vi "load user configuration.vi"() -> (1 "RT config file path":path, 3 "config parameters":T13 {"messageHandler"."params"."controlChannels"."ballControl" items=["Module6/output0", "Module6/output1", "Module6/output2", "Module6/output3", "Not-Used"]; "messageHandler"."params"."controlChannels"."butterflyControl" items=["Module6/output0", "Module6/output1", "Module6/output2", "Module6/output3", "Not-Used"]; "messageHandler"."params"."controlChannels"."speedControl" items=["Module6/output0", "Module6/output1", "Module6/output2", "Module6/output3", "Not-Used"]})   [LabVIEW 2018]
uses:
  type defs/message handler data.ctl
  customVI/liveData/state.ctl
  type defs/comms loop data.ctl
  ICL-LabVIEW_General/Incident logger/Incident logger.lvclass
  <vilib>/Modbus/master/Modbus Master.lvclass
  type defs/data stream data.ctl
  type defs/data processor data.ctl
  type defs/channelLimitControl.ctl
  type defs/limitActions.ctl
  type defs/file IO data.ctl
  type defs/channelControl.ctl
  RT/Type Defs/channelScalingTypes.ctl
  RT/Type Defs/scalingMethods.ctl
  ICL-LabVIEW_General/data channels/parent class/Data Channel.lvclass
  type defs/UI loop data.ctl
  type defs/error messages data.ctl
  <vilib>/Utility/config.llb/Read Key (Path).vi
  <vilib>/Utility/config.llb/Read Key (U32).vi
  <vilib>/Utility/config.llb/Read Key (Boolean).vi
  <vilib>/Utility/config.llb/Read Key (Double).vi
  <vilib>/Utility/config.llb/Read Key (String).vi
  <vilib>/Utility/config.llb/NI_LVConfig.lvlib
panel:
  out "Default parameters":string[](array[string])
  out "unmatched parameters":string[](array[string])
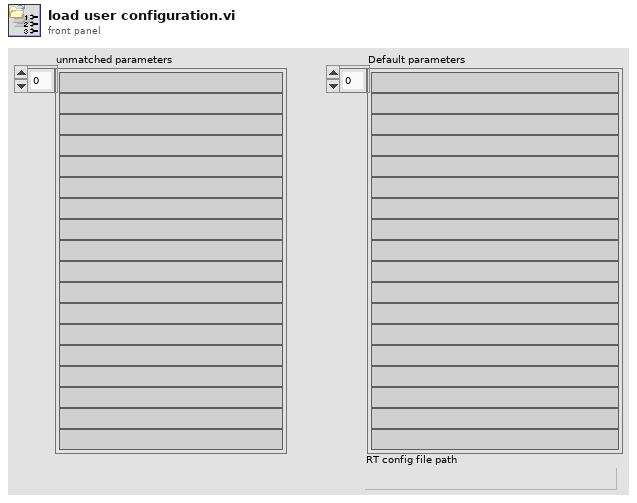
[diagram p1: front panel]
types:
  T1 = typedef "message handler data.ctl" = cluster{"params":cluster{"configFileID":u32, "configFilePath":path, "channelConfigFilePath":path, "incidentLogfile":path, "controlChannels":cluster{"ballControl":u16, "butterflyControl":u16, "speedControl":u16}, "pulsatorVIPath":path, "customVIPath":path, "HowdenAir":cluster{"vent Howden":bool, "Howden%":dbl}}, "vars":cluster{"commsStatus":bool[], "controlIndex":cluster{"ballControl":u16, "butterflyControl":u16, "speedControl":u16}, "customVIRef":refnum<vi>, "Interlocks":cluster{"gearboxOil":bool, "bearingOil":bool, "gearboxAir":bool}, "motorRunning":bool, "liveDataQ":refnum<queue>[]}}
  T2 = typedef "comms loop data.ctl" = cluster{"params":cluster{"commandStream":cluster{"reader name":string, "writer name":string, "stream buffer size":i32}, "errorStream":cluster{"reader name":string, "writer name":string, "stream buffer size":i32}, "RT IP address":string, "pulserControllerIP":string}, "vars":cluster{"commandStream":refnum<k21>, "Incident logger":refnum<class "Incident logger.lvclass">, "check error scheduled message":u32, "errorStream":refnum<k21>, "watchdogScheduleID":u32, "pulsator":cluster{"pulser connection":refnum<class "Modbus Master.lvclass">, "pulserConnected":bool, "pulsatorScheduleID":u32, "pulserRunning":bool}}}
  T3 = typedef "data stream data.ctl" = cluster{"params":cluster{"Stream":cluster{"reader name":string, "RT IP address":string, "writer name":string, "stream buffer size":i32}}, "vars":cluster{"data stream":refnum<k21>}}
  T4 = typedef "data processor data.ctl" = cluster{"params":cluster{"controlFeedback":cluster{"butterflyValue":u16, "ballValue":u16, "massflow":u16, "pressureRatio":u16, "compSpeed":u16}, "DAQrate":enum16{"50 kHz", "25 kHz", "16.6 kHz", "12.5 kHz", "10 kHz", "8.33 kHz", "7.14 kHz", "6.25 kHz", "5.55 kHz", "5 kHz"}, "safetyChannels":cluster{"oilP":u16, "airP":u16, "water":u16, "channelLimit":T5[]}, "channelConfigPath":path}, "vars":cluster{"controlFeedback":cluster{"butterflyValue":u16, "ballValue":u16, "massflow":u16, "pressureRatio":u16, "compSpeed":u16}, "activeChannelNames":string[], "activeChannelUnits":string[], "offset trigger":bool, "offsets":dbl[], "activeChannelLimitIndex":u16[], "liveData":bool}}
  T5 = typedef "channelLimitControl.ctl" = cluster{"channelID":u16, "Enabled":bool, "warnValue":dbl, "limitValue":dbl, "Invert":bool, "limitAction":T6}
  T6 = typedef "limitActions.ctl" = enum16{"stop", "shutdown", "ignore"}
  T7 = typedef "file IO data.ctl" = cluster{"params":cluster{"startFolder":path, "channelConfigPath":path}, "vars":cluster{"channelConfig ":T8[], "writing":cluster{"streaming":bool, "fixedLength":bool, "pointCount":u32, "timeZero":dbl, "pointsWritten":u32, "dataRate":u16}, "channelCount":u16, "fileTarget":cluster{"Save folder":path, "Target filename":string, "file ref":refnum<file>, "pulsatorSpeed":string, "motorSpeed":string, "valvePosition":string, "torqueFilter":bool, "pulsatorRunning":bool, "motorRunning":bool}, "channels":refnum<class "Data Channel.lvclass">[]}}
  T8 = typedef "channelControl.ctl" = cluster{"index":u16, "active":bool, "channelType":T9, "module":u16, "terminal":u16, "channelName":string, "scalingMethod":T10, "scalingParameters":dbl[], "scaledUnits":string, "tempOffset":dbl}
  T9 = typedef "channelScalingTypes.ctl" = enum16{"calculation", "measurement", "scanivalve", "output", "digital"}
  T10 = typedef "scalingMethods.ctl" = enum16{"none", "linear", "thermocouple", "polynomial", "encoder", "RTD"}
  T11 = typedef "UI loop data.ctl" = cluster{"params":cluster{"channelConfigPath":path, "version":string}, "vars":cluster{"tempOffsets":dbl[], "encoderFallingEdge":bool, "controlRefs":cluster{"mainVI":refnum<vi>, "menu":refnum<k9>, "motorStart":refnum<vi>, "butterfly":refnum<vi>, "ball":refnum<vi>, "speed":refnum<vi>, "logLimit":refnum<vi>, "pointLimit":refnum<vi>, "logData":refnum<vi>}}}
  T12 = typedef "error messages data.ctl" = cluster{"params":cluster{"eg":bool}, "vars":cluster{"eg":bool}}
  T13 = cluster{"messageHandler":T1, "comms":T2, "dataStream":T3, "dataProcessor":T4, "fileIO":T7, "userInterface":T11, "errors":T12}
  T14 = typedef "NI_LVConfig.lvlib/Config Data RefNum.ctl" = refnum<k1>
  T15 = typedef "Message loop data.ctl" = cluster{"Parameters":cluster{"FPGA Ref":T16, "configID":u32, "activeChannels":cluster{"index":u16, "name":string}[]}, "Variables":cluster{"RT Status":T17, "watchdog":timestamp, "limitsEnabled":bool, "Interlocks":cluster{"gearboxOil":bool, "bearingOil":bool, "gearboxAir":bool}}}
  T16 = typedef "FPGA reference.ctl" = refnum<k20>
  T17 = typedef "RT Status.ctl" = cluster{"Comms loop":bool, "scheduler loop":bool, "data process loop":bool, "FIFO loop":bool, "Command Stream":bool, "Error Stream":bool, "FPGA FIFO":bool, "Data Stream":bool}
  T18 = typedef "Analogue loop data.ctl" = cluster{"Params":cluster{"FPGA ref":T16, "Total Channels":u32}, "Variables":cluster{"FIFO wait counter":u16, "FIFO read trigger":u32}}
  T19 = typedef "comms data.ctl" = cluster{"Parameters":cluster{"error writer name":string, "command reader name":string, "error buffer size":i32, "command buffer size":i32, "scanivalveIP":string, "scanivalvePeriod":u16}, "Variables":cluster{"listen schedule":u32, "incident buffer":T20[], "command stream":refnum<k21>, "error stream":refnum<k21>, "waiting for command stream connect":bool, "waiting for error stream connect":bool, "scanivalve connection":refnum<k5>, "scanivalveScheduleID":u32, "activeScanivalvePorts":i32[], "channelCount":i16}, "scanivalveConfig":T21}
  T20 = typedef "generic incident.ctl" = cluster{"timestamp":timestamp, "type":string, "Variant":variant}
  T21 = typedef "Scanivalve API.lvlib/scanivalveConfig.ctl" = cluster{"listS":T22, "listC":T23, "listSG":T24, "activeChannels":T25}
  T22 = typedef "Scanivalve API.lvlib/listS.ctl" = cluster{"period":u16, "ADtrig":bool, "ScanTrig":bool, "page":u16, "qpkts":u16}
  T23 = typedef "Scanivalve API.lvlib/listC.ctl" = cluster{"ZC":bool, "unitScan":string, "CvtUnit":dbl, "bin":bool, "EU":bool}
  T24 = typedef "Scanivalve API.lvlib/listSG.ctl" = cluster{"Avg1":u16, "FPS1":u16, "SGEnable1":bool}
  T25 = typedef "Scanivalve API.lvlib/chan1.ctl" = cluster{"Chan1":cluster{"101":bool, "102":bool, "103":bool, "104":bool, "109":bool, "110":bool, "111":bool, "112":bool, "201":bool, "202":bool, "203":bool, "204":bool, "209":bool, "210":bool, "211":bool, "212":bool, "301":bool, "302":bool, "303":bool, "304":bool, "309":bool, "310":bool, "311":bool, "312":bool, "401":bool, "402":bool, "403":bool, "404":bool, "409":bool, "410":bool, "411":bool, "412":bool}}
  T26 = typedef "Data processing loop data.ctl" = cluster{"Parameters":cluster{"FPGA Ref":T16, "data stream":cluster{"data writer name":string, "NS write buffer size":i32, "NS Buffer length":u32}, "FIFO Depth":u32, "Channel controls":cluster{"FIFO channel count":i32, "active indices":i16[], "active channels":i32, "channelScaling":T8[], "scanivalveCount":i32, "channels":refnum<class "Data Channel.lvclass">[]}, "safetyChannels":cluster{"oilP":u16, "airP":u16, "water":u16, "channelLimits":T5[]}, "speedChannel":i32, "maxSpeedLimit":dbl, "Torque":cluster{"fixedOffset":dbl, "filter":bool, "fallingEdge":bool, "swapEncoders":bool}}, "Variables":cluster{"Intermediary buffer":dbl[][], "buffer position":u32, "write loop counter":u16, "NS write trigger":u32, "NS Connection status":bool, "waiting for NS":bool, "labAmbient":cluster{"pressure":dbl, "temperature":dbl}, "scanivalvePorts":u16[], "scanivalvePressures":dbl[], "data stream":refnum<k21>, "activeChannelLimitIndex":u16[], "runningSpeedLimit":dbl, "speedChannelIndex":i32, "Interlocks":cluster{"gearboxOil":bool, "bearingOil":bool, "gearboxAir":bool}, "interlockChannels":cluster{"gearboxOil":i32, "bearingOil":i32, "air":i32}, "limitStates":cluster{"warn":bool, "alarm":bool}[]}}
  T27 = cluster{"Message":T15, "FIFO":T18, "Comms data":T19, "Data processor":T26}
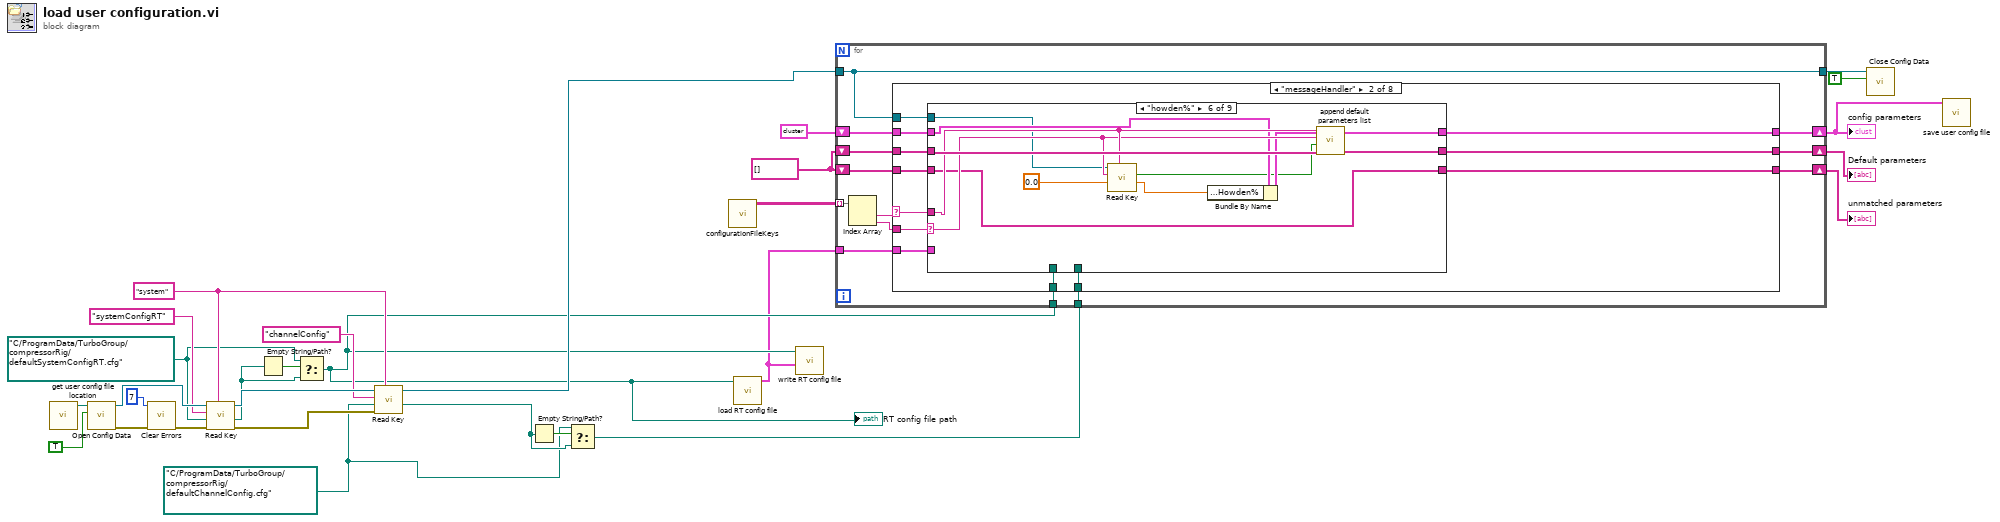
[diagram p0: block diagram]
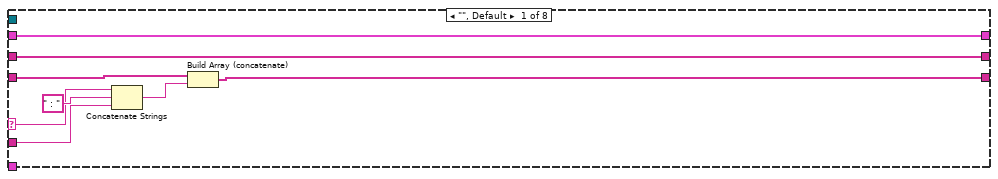
[diagram p2: hidden frame]
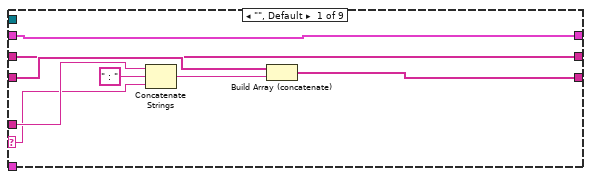
[diagram p3: hidden frame]
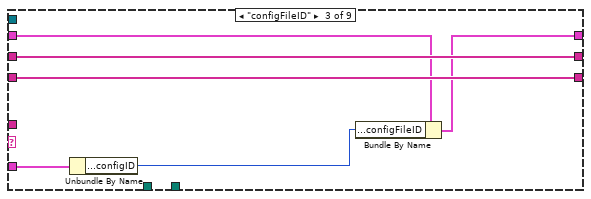
[diagram p5: hidden frame]
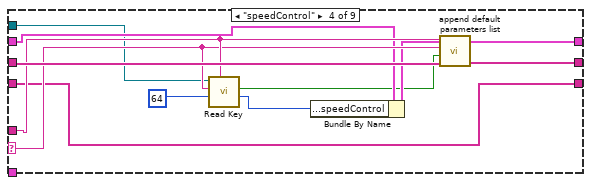
[diagram p6: hidden frame]
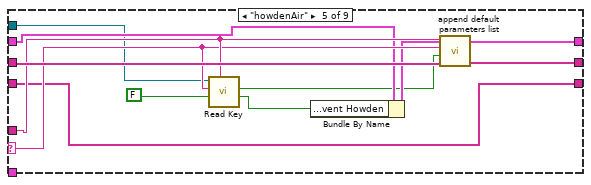
[diagram p7: hidden frame]
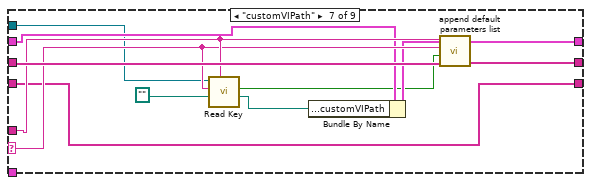
[diagram p8: hidden frame]
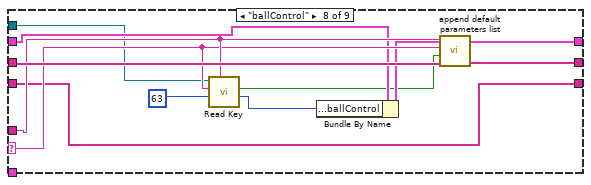
[diagram p9: hidden frame]
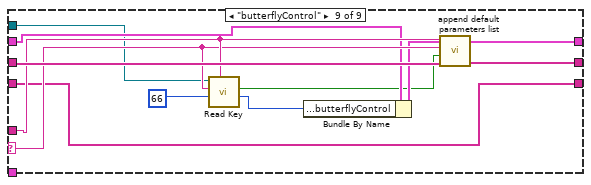
[diagram p10: hidden frame]
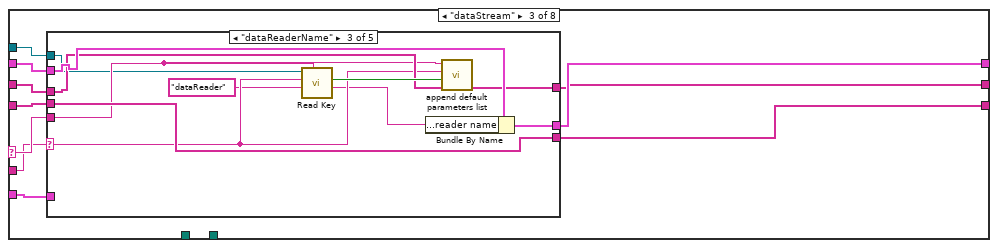
[diagram p11: hidden frame]
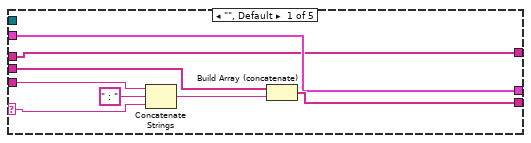
[diagram p12: hidden frame]
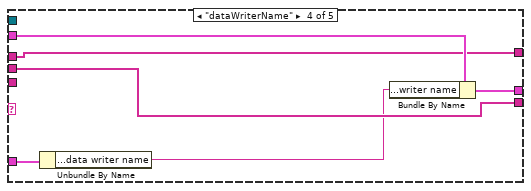
[diagram p14: hidden frame]
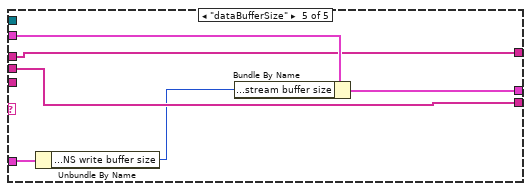
[diagram p15: hidden frame]
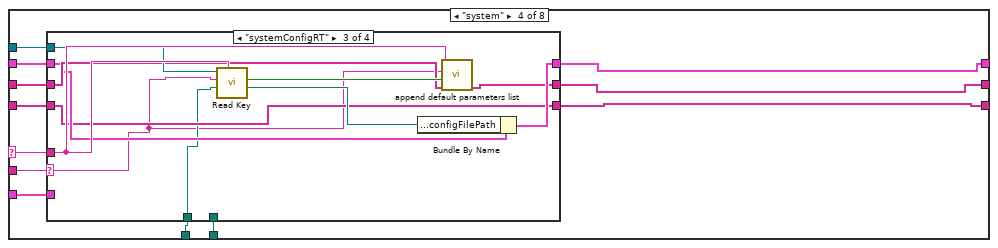
[diagram p16: hidden frame]
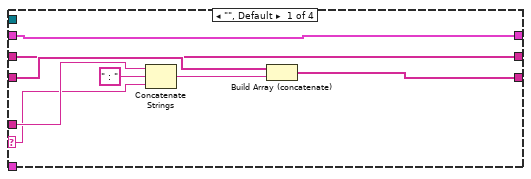
[diagram p17: hidden frame]
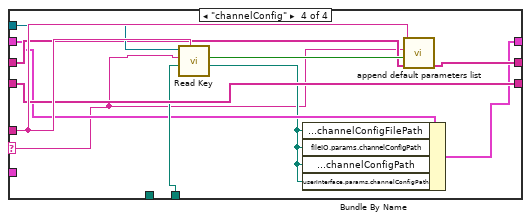
[diagram p19: hidden frame]
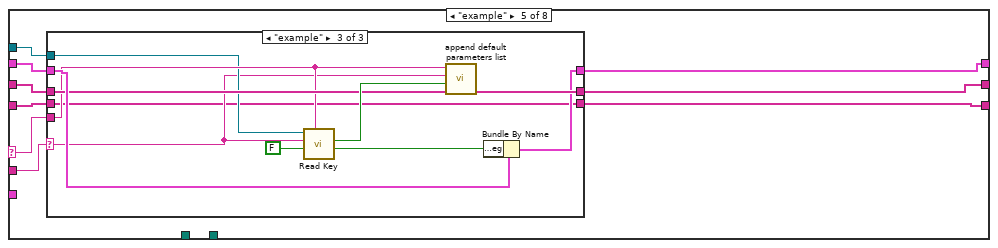
[diagram p20: hidden frame]
diagram:
  w20 = string[] []
  w4 = path "C:/ProgramData/TurboGroup/compressorRig/defaultChannelConfig.cfg" ("default value")
  w7 = path "C:/ProgramData/TurboGroup/compressorRig/defaultSystemConfigRT.cfg" ("default value")
  w23 = "system" ("section")
  n1 = call "get user config file location.vi"() -> ("userConfigPath"=w29:path)  [unwired: 11 in]
  n2 = call <vilib>:"Open Config Data.vi"("create file if necessary (T)"=TRUE, "configuration file path"=w29) -> ("error out"=w27:errorcluster, "refnum"=w28:T14)  [unwired: 7 in, 1 out]
  n3 = call <vilib>:"Clear Errors.vi"("error in (no error)"=w27, "specific error code to clear (0: all)"=7) -> ("error out"=w14:errorcluster)  [unwired: 4 in, 1 out]
  n4 = call-poly <vilib>:"Read Key.vi"("section"=w23, "error in (no error)"=w14, "default value"=w7, "key"="systemConfigRT", "refnum"=w28) -> ("error out"=w24:errorcluster, "value"=w8:path, "refnum out"=w25:T14)  [unwired: 3 in, 1 out]
  n5 = Empty String/Path?(string/path=w8) -> (empty?=w9:bool)
  n6 = Select(t=w7, s=w9, f=w8) -> (s? t:f=w2:path)
  "RT config file path" <- w2
  n7 = call-poly <vilib>:"Read Key.vi"("section"=w23, "error in (no error)"=w24, "default value"=w4, "key"="channelConfig", "refnum"=w25) -> ("value"=w5:path, "refnum out"=w18:T14)  [unwired: 3 in, 2 out]
  n8 = Empty String/Path?(string/path=w5) -> (empty?=w6:bool)
  n9 = Select(t=w4, s=w6, f=w5) -> (s? t:f=w3:path)
  n10 = call "configurationFileKeys.vi"() -> ("userConfigKeys"=w16:string[][])  [unwired: 9 in, 2 out]
  n11 = call "load RT config file.vi"("configuration file path (RT local)"=w2) -> ("config data out"=w1:T27)  [unwired: 7 in, 3 out]
  n12 = call "write RT config file.vi"("RT config"=w1, "RT config file path"=w2) -> ()  [unwired: 10 in]
  n13 = for {
    shift-right: [w41] -> w21
    shift-left: w20 -> [w42]
    shift-right: [w39] -> w10
    shift-left: T13 {"messageHandler"={"params"={"configFileID"=0, "configFilePath"=path "", "channelConfigFilePath"=path "", "incidentLogfile"=path "", "controlChannels"={"ballControl"=0, "butterflyControl"=0, "speedControl"=0}, "pulsatorVIPath"=path "", "customVIPath"=path "", "HowdenAir"={"vent Howden"=FALSE, "Howden%"=0.0}}, "vars"={"commsStatus"=[], "controlIndex"={"ballControl"=0, "butterflyControl"=0, "speedControl"=0}, "customVIRef"=refnum, "Interlocks"={"gearboxOil"=FALSE, "bearingOil"=FALSE, "gearboxAir"=FALSE}, "motorRunning"=FALSE, "liveDataQ"=[]}}, "comms"={"params"={"commandStream"={"reader name"="", "writer name"="", "stream buffer size"=0}, "errorStream"={"reader name"="", "writer name"="", "stream buffer size"=0}, "RT IP address"="", "pulserControllerIP"=""}, "vars"={"commandStream"="", "Incident logger"=refnum, "check error scheduled message"=0, "errorStream"="", "watchdogScheduleID"=0, "pulsator"={"pulser connection"=refnum, "pulserConnected"=FALSE, "pulsatorScheduleID"=0, "pulserRunning"=FALSE}}}, "dataStream"={"params"={"Stream"={"reader name"="", "RT IP address"="", "writer name"="", "stream buffer size"=0}}, "vars"={"data stream"=""}}, "dataProcessor"={"params"={"controlFeedback"={"butterflyValue"=0, "ballValue"=0, "massflow"=0, "pressureRatio"=0, "compSpeed"=0}, "DAQrate"=enum."50 kHz", "safetyChannels"={"oilP"=0, "airP"=0, "water"=0, "channelLimit"=[]}, "channelConfigPath"=path ""}, "vars"={"controlFeedback"={"butterflyValue"=0, "ballValue"=0, "massflow"=0, "pressureRatio"=0, "compSpeed"=0}, "activeChannelNames"=[], "activeChannelUnits"=[], "offset trigger"=FALSE, "offsets"=[], "activeChannelLimitIndex"=[], "liveData"=FALSE}}, "fileIO"={"params"={"startFolder"=path "", "channelConfigPath"=path ""}, "vars"={"channelConfig "=[], "writing"={"streaming"=FALSE, "fixedLength"=FALSE, "pointCount"=0, "timeZero"=0.0, "pointsWritten"=0, "dataRate"=0}, "channelCount"=0, "fileTarget"={"Save folder"=path "", "Target filename"="", "file ref"=refnum, "pulsatorSpeed"="", "motorSpeed"="", "valvePosition"="", "torqueFilter"=FALSE, "pulsatorRunning"=FALSE, "motorRunning"=FALSE}, "channels"=[]}}, "userInterface"={"params"={"channelConfigPath"=path "", "version"=""}, "vars"={"tempOffsets"=[], "encoderFallingEdge"=FALSE, "controlRefs"={"mainVI"=refnum, "menu"=refnum, "motorStart"=refnum, "butterfly"=refnum, "ball"=refnum, "speed"=refnum, "logLimit"=refnum, "pointLimit"=refnum, "logData"=refnum}}}, "errors"={"params"={"eg"=FALSE}, "vars"={"eg"=FALSE}}} ("parameters") -> [w40]
    tunnel: w18 -> [w33]
    tunnel: w16 -> [w38] mode=indexing
    shift-right: [w35] -> w19
    shift-left: w20 -> [w34]
    tunnel: [w33] -> w15
    tunnel: w1 -> [w32]
    tunnel: w2 -> [w31]
    tunnel: w3 -> [w30]
    n14 = Index Array(array=w38) -> (element #1=w37:string, element #2=w36:string)  [unwired: 2 in]
    n15 = case shown="\"messageHandler\"" w37 {
      selector: w37 -> [w46 w61 w154 w194 w242 w273 w370 w402]
      tunnel: w42 -> [w48 w62 w155 w198 w243 w274 w371 w403]
      tunnel: [w47 w60 w153 w196 w241 w272 w369 w401] -> w41
      tunnel: w40 -> [w45 w58 w151 w200 w239 w270 w367 w400]
      tunnel: [w45 w59 w152 w201 w240 w271 w368 w399] -> w39
      tunnel: w33 -> [_ w54 w147 w195 w235 w266 w363 w398]
      tunnel: w36 -> [w44 w57 w150 w193 w238 w269 w366 w397]
      tunnel: [w43 w56 w149 w197 w237 w268 w365 w395] -> w35
      tunnel: w34 -> [w43 w55 w148 w199 w236 w267 w364 w396]
      tunnel: w32 -> [_ w53 w146 w192 _ _ _ w394]
      tunnel: w31 -> [_ w52 _ w191 _ _ _ _]
      tunnel: w30 -> [_ w51 _ w190 _ _ _ _]
      frame "", Default {
        n16 = Concatenate Strings(w46, " : " ("string"), w44) -> (w49:string)
        n17 = Build Array (concatenate)(w48, w49) -> (w47:string[])
      }
      frame "messageHandler" {
        n18 = case shown="\"howden%\"" w57 {
          selector: w57 -> [w68 _ _ w87 w98 w109 w120 w131 w142]
          tunnel: w62 -> [w70 w73 w79 w84 w96 w107 w118 w128 w139]
          tunnel: w61 -> [w69 _ _ w88 w99 w110 w121 w132 w143]
          tunnel: [w65 w73 w79 w84 w96 w107 w118 w128 w139] -> w60
          tunnel: [w64 w72 w75 w83 w95 w106 w117 w127 w138] -> w59
          tunnel: w58 -> [w64 w72 w76 w85 w97 w108 w119 w129 w140]
          tunnel: [w63 w71 w78 w90 w101 w112 w123 w134 w145] -> w56
          tunnel: w55 -> [w63 w71 w78 w89 w100 w111 w122 w133 w144]
          tunnel: w54 -> [_ _ _ w80 w92 w103 w114 w124 w135]
          tunnel: w53 -> [_ _ w77 _ _ _ _ _ _]
          tunnel: w52 -> [_ _ _ _ _ _ _ _ _]
          tunnel: w51 -> [_ _ _ _ _ _ _ _ _]
          frame "", Default {
            n19 = Concatenate Strings(w69, " : " ("string"), w68) -> (w66:string)
            n20 = Build Array (concatenate)(w70, w66) -> (w65:string[])
          }
          frame "none" {
          }
          frame "configFileID" {
            n21 = Unbundle By Name(w77) -> ("Message.Parameters.configID"=w74:u32)
            n22 = Bundle By Name(cluster=w76, "messageHandler.params.configFileID"=w74) -> (w75:T13)
          }
          frame "speedControl" {
            n23 = call-poly <vilib>:"Read Key.vi"("section"=w88, "default value"=u16 64, "key"=w87, "refnum"=w80) -> ("value"=w82:u32, "found?"=w81:bool)  [unwired: 4 in, 2 out]
            n24 = Bundle By Name(cluster=w85, "messageHandler.params.controlChannels.speedControl"=w82) -> (w83:T13)
            n25 = call "append default parameters list.vi"("default parameters in"=w89, "parameter found?"=w81, "Key"=w87, "Section"=w88) -> ("default parameters out"=w90:string[])  [unwired: 7 in]
          }
          frame "howdenAir" {
            n26 = call-poly <vilib>:"Read Key.vi"("section"=w99, "default value"=FALSE, "key"=w98, "refnum"=w92) -> ("value"=w94:bool, "found?"=w93:bool)  [unwired: 4 in, 2 out]
            n27 = Bundle By Name(cluster=w97, "messageHandler.params.HowdenAir.vent Howden"=w94) -> (w95:T13)
            n28 = call "append default parameters list.vi"("default parameters in"=w100, "parameter found?"=w93, "Key"=w98, "Section"=w99) -> ("default parameters out"=w101:string[])  [unwired: 7 in]
          }
          frame "howden%" {
            n29 = call-poly <vilib>:"Read Key.vi"("section"=w110, "default value"=0.0, "key"=w109, "refnum"=w103) -> ("value"=w105:dbl, "found?"=w104:bool)  [unwired: 4 in, 2 out]
            n30 = Bundle By Name(cluster=w108, "messageHandler.params.HowdenAir.Howden%"=w105) -> (w106:T13)
            n31 = call "append default parameters list.vi"("default parameters in"=w111, "parameter found?"=w104, "Key"=w109, "Section"=w110) -> ("default parameters out"=w112:string[])  [unwired: 7 in]
          }
          frame "customVIPath" {
            n32 = call-poly <vilib>:"Read Key.vi"("section"=w121, "default value"=path "", "key"=w120, "refnum"=w114) -> ("value"=w116:path, "found?"=w115:bool)  [unwired: 4 in, 2 out]
            n33 = Bundle By Name(cluster=w119, "messageHandler.params.customVIPath"=w116) -> (w117:T13)
            n34 = call "append default parameters list.vi"("default parameters in"=w122, "parameter found?"=w115, "Key"=w120, "Section"=w121) -> ("default parameters out"=w123:string[])  [unwired: 7 in]
          }
          frame "ballControl" {
            n35 = call-poly <vilib>:"Read Key.vi"("section"=w132, "default value"=u16 63, "key"=w131, "refnum"=w124) -> ("value"=w126:u32, "found?"=w125:bool)  [unwired: 4 in, 2 out]
            n36 = Bundle By Name(cluster=w129, "messageHandler.params.controlChannels.ballControl"=w126) -> (w127:T13)
            n37 = call "append default parameters list.vi"("default parameters in"=w133, "parameter found?"=w125, "Key"=w131, "Section"=w132) -> ("default parameters out"=w134:string[])  [unwired: 7 in]
          }
          frame "butterflyControl" {
            n38 = call-poly <vilib>:"Read Key.vi"("section"=w143, "default value"=u16 66, "key"=w142, "refnum"=w135) -> ("value"=w137:u32, "found?"=w136:bool)  [unwired: 4 in, 2 out]
            n39 = Bundle By Name(cluster=w140, "messageHandler.params.controlChannels.butterflyControl"=w137) -> (w138:T13)
            n40 = call "append default parameters list.vi"("default parameters in"=w144, "parameter found?"=w136, "Key"=w142, "Section"=w143) -> ("default parameters out"=w145:string[])  [unwired: 7 in]
          }
        }
      }
      frame "dataStream" {
        n41 = case shown="\"dataReaderName\"" w150 {
          selector: w150 -> [w161 _ w170 _ _]
          tunnel: w155 -> [w163 w166 w177 w183 w189]
          tunnel: w154 -> [w162 _ w171 _ _]
          tunnel: [w158 w166 w177 w183 w189] -> w153
          tunnel: [w157 w165 w175 w181 w187] -> w152
          tunnel: w151 -> [w157 w165 w176 w182 w188]
          tunnel: [w156 w164 w172 w178 w184] -> w149
          tunnel: w148 -> [w156 w164 w173 w178 w184]
          tunnel: w147 -> [_ _ w169 _ _]
          tunnel: w146 -> [_ _ _ w180 w186]
          frame "", Default {
            n42 = Concatenate Strings(w162, " : " ("string"), w161) -> (w159:string)
            n43 = Build Array (concatenate)(w163, w159) -> (w158:string[])
          }
          frame "none" {
          }
          frame "dataReaderName" {
            n44 = call-poly <vilib>:"Read Key.vi"("section"=w171, "default value"="dataReader" ("name or relative path"), "key"=w170, "refnum"=w169) -> ("value"=w167:string, "found?"=w174:bool)  [unwired: 4 in, 2 out]
            n45 = Bundle By Name(cluster=w176, "dataStream.params.Stream.reader name"=w167) -> (w175:T13)
            n46 = call "append default parameters list.vi"("default parameters in"=w173, "parameter found?"=w174, "Key"=w170, "Section"=w171) -> ("default parameters out"=w172:string[])  [unwired: 7 in]
          }
          frame "dataWriterName" {
            n47 = Unbundle By Name(w180) -> ("Data processor.Parameters.data stream.data writer name"=w179:string)
            n48 = Bundle By Name(cluster=w182, "dataStream.params.Stream.writer name"=w179) -> (w181:T13)
          }
          frame "dataBufferSize" {
            n49 = Unbundle By Name(w186) -> ("Data processor.Parameters.data stream.NS write buffer size"=w185:i32)
            n50 = Bundle By Name(cluster=w188, "dataStream.params.Stream.stream buffer size"=w185) -> (w187:T13)
          }
        }
      }
      frame "system" {
        n51 = case shown="\"systemConfigRT\"" w193 {
          selector: w193 -> [w207 _ w213 w224]
          tunnel: w198 -> [w209 w212 w216 w230]
          tunnel: w194 -> [w208 _ w221 w233]
          tunnel: [w204 w212 w216 w230] -> w196
          tunnel: [w203 w211 w217 w226] -> w201
          tunnel: w200 -> [w203 w211 w218 w227]
          tunnel: [w202 w210 w215 w229] -> w197
          tunnel: w199 -> [w202 w210 w219 w231]
          tunnel: w195 -> [_ _ w220 w232]
          tunnel: w192 -> [_ _ _ _]
          tunnel: w191 -> [_ _ w214 _]
          tunnel: w190 -> [_ _ _ w228]
          frame "", Default {
            n52 = Concatenate Strings(w208, " : " ("string"), w207) -> (w205:string)
            n53 = Build Array (concatenate)(w209, w205) -> (w204:string[])
          }
          frame "none" {
          }
          frame "systemConfigRT" {
            n54 = call-poly <vilib>:"Read Key.vi"("section"=w221, "default value"=w214, "key"=w213, "refnum"=w220) -> ("value"=w222:path, "found?"=w223:bool)  [unwired: 4 in, 2 out]
            n55 = Bundle By Name(cluster=w218, "messageHandler.params.configFilePath"=w222) -> (w217:T13)
            n56 = call "append default parameters list.vi"("default parameters in"=w219, "parameter found?"=w223, "Key"=w213, "Section"=w221) -> ("default parameters out"=w215:string[])  [unwired: 7 in]
          }
          frame "channelConfig" {
            n57 = call-poly <vilib>:"Read Key.vi"("section"=w233, "default value"=w228, "key"=w224, "refnum"=w232) -> ("value"=w225:path, "found?"=w234:bool)  [unwired: 4 in, 2 out]
            n58 = Bundle By Name(cluster=w227, "messageHandler.params.channelConfigFilePath"=w225, "fileIO.params.channelConfigPath"=w225, "dataProcessor.params.channelConfigPath"=w225, "userInterface.params.channelConfigPath"=w225) -> (w226:T13)
            n59 = call "append default parameters list.vi"("default parameters in"=w231, "parameter found?"=w234, "Key"=w224, "Section"=w233) -> ("default parameters out"=w229:string[])  [unwired: 7 in]
          }
        }
      }
      frame "example" {
        n60 = case shown="\"example\"" w238 {
          selector: w238 -> [w249 _ w256]
          tunnel: w243 -> [w251 w254 w255]
          tunnel: w242 -> [w250 _ w258]
          tunnel: [w246 w254 w255] -> w241
          tunnel: [w245 w253 w260] -> w240
          tunnel: w239 -> [w245 w253 w261]
          tunnel: [w244 w252 w262] -> w237
          tunnel: w236 -> [w244 w252 w259]
          tunnel: w235 -> [_ _ w257]
          frame "", Default {
            n61 = Concatenate Strings(w250, " : " ("string"), w249) -> (w247:string)
            n62 = Build Array (concatenate)(w251, w247) -> (w246:string[])
          }
          frame "none" {
          }
          frame "example" {
            n63 = call-poly <vilib>:"Read Key.vi"("section"=w258, "default value"=FALSE, "key"=w256, "refnum"=w257) -> ("value"=w264:bool, "found?"=w265:bool)  [unwired: 4 in, 2 out]
            n64 = call "append default parameters list.vi"("default parameters in"=w259, "parameter found?"=w265, "Key"=w256, "Section"=w258) -> ("default parameters out"=w262:string[])  [unwired: 7 in]
            n65 = Bundle By Name(cluster=w261, "errors.params.eg"=w264) -> (w260:T13)
          }
        }
      }
      frame "dataProcessor" {
        n66 = case shown="\"totalChannels\"" w269 {
          selector: w269 -> [w280 _ w289 w300 w311 w322 w333 w344 w355]
          tunnel: w274 -> [w282 w285 w288 w299 w310 w321 w332 w343 w354]
          tunnel: w273 -> [w281 _ w291 w302 w313 w324 w335 w346 w357]
          tunnel: [w277 w285 w288 w299 w310 w321 w332 w343 w354] -> w272
          tunnel: [w276 w284 w293 w304 w315 w326 w337 w348 w359] -> w271
          tunnel: w270 -> [w276 w284 w294 w305 w316 w327 w338 w349 w360]
          tunnel: [w275 w283 w295 w306 w317 w328 w339 w350 w361] -> w268
          tunnel: w267 -> [w275 w283 w292 w303 w314 w325 w336 w347 w358]
          tunnel: w266 -> [_ _ w290 w301 w312 w323 w334 w345 w356]
          frame "", Default {
            n67 = Concatenate Strings(w281, " : " ("string"), w280) -> (w278:string)
            n68 = Build Array (concatenate)(w282, w278) -> (w277:string[])
          }
          frame "none" {
          }
          frame "butterflyChannel" {
            n69 = call-poly <vilib>:"Read Key.vi"("section"=w291, "default value"=u16 49 ("dataProcessor.params.controlFeedback.butterflyValue"), "key"=w289, "refnum"=w290) -> ("value"=w286:u32, "found?"=w296:bool)  [unwired: 4 in, 2 out]
            n70 = call "append default parameters list.vi"("default parameters in"=w292, "parameter found?"=w296, "Key"=w289, "Section"=w291) -> ("default parameters out"=w295:string[])  [unwired: 7 in]
            n71 = Bundle By Name(cluster=w294, "dataProcessor.params.controlFeedback.butterflyValue"=w286, "messageHandler.params.controlChannels.butterflyControl"=w286) -> (w293:T13)
          }
          frame "ballChannel" {
            n72 = call-poly <vilib>:"Read Key.vi"("section"=w302, "default value"=u16 50 ("dataProcessor.params.controlFeedback.butterflyValue"), "key"=w300, "refnum"=w301) -> ("value"=w297:u32, "found?"=w307:bool)  [unwired: 4 in, 2 out]
            n73 = call "append default parameters list.vi"("default parameters in"=w303, "parameter found?"=w307, "Key"=w300, "Section"=w302) -> ("default parameters out"=w306:string[])  [unwired: 7 in]
            n74 = Bundle By Name(cluster=w305, "dataProcessor.params.controlFeedback.ballValue"=w297, "messageHandler.params.controlChannels.ballControl"=w297) -> (w304:T13)
          }
          frame "massflow" {
            n75 = call-poly <vilib>:"Read Key.vi"("section"=w313, "default value"=u16 104 ("dataProcessor.params.controlFeedback.butterflyValue"), "key"=w311, "refnum"=w312) -> ("value"=w308:u32, "found?"=w318:bool)  [unwired: 4 in, 2 out]
            n76 = call "append default parameters list.vi"("default parameters in"=w314, "parameter found?"=w318, "Key"=w311, "Section"=w313) -> ("default parameters out"=w317:string[])  [unwired: 7 in]
            n77 = Bundle By Name(cluster=w316, "dataProcessor.params.controlFeedback.massflow"=w308) -> (w315:T13)
          }
          frame "pressureRatio" {
            n78 = call-poly <vilib>:"Read Key.vi"("section"=w324, "default value"=u16 20 ("dataProcessor.params.controlFeedback.butterflyValue"), "key"=w322, "refnum"=w323) -> ("value"=w319:u32, "found?"=w329:bool)  [unwired: 4 in, 2 out]
            n79 = call "append default parameters list.vi"("default parameters in"=w325, "parameter found?"=w329, "Key"=w322, "Section"=w324) -> ("default parameters out"=w328:string[])  [unwired: 7 in]
            n80 = Bundle By Name(cluster=w327, "dataProcessor.params.controlFeedback.pressureRatio"=w319) -> (w326:T13)
          }
          frame "speedChannel" {
            n81 = call-poly <vilib>:"Read Key.vi"("section"=w335, "default value"=u16 59 ("dataProcessor.params.controlFeedback.butterflyValue"), "key"=w333, "refnum"=w334) -> ("value"=w330:u32, "found?"=w340:bool)  [unwired: 4 in, 2 out]
            n82 = call "append default parameters list.vi"("default parameters in"=w336, "parameter found?"=w340, "Key"=w333, "Section"=w335) -> ("default parameters out"=w339:string[])  [unwired: 7 in]
            n83 = Bundle By Name(cluster=w338, "dataProcessor.params.controlFeedback.compSpeed"=w330, "messageHandler.params.controlChannels.speedControl"=w330) -> (w337:T13)
          }
          frame "oilPressure" {
            n84 = call-poly <vilib>:"Read Key.vi"("section"=w346, "default value"=u16 59 ("dataProcessor.params.controlFeedback.butterflyValue"), "key"=w344, "refnum"=w345) -> ("value"=w341:u32, "found?"=w351:bool)  [unwired: 4 in, 2 out]
            n85 = call "append default parameters list.vi"("default parameters in"=w347, "parameter found?"=w351, "Key"=w344, "Section"=w346) -> ("default parameters out"=w350:string[])  [unwired: 7 in]
            n86 = Bundle By Name(cluster=w349, "dataProcessor.params.safetyChannels.oilP"=w341) -> (w348:T13)
          }
          frame "totalChannels" {
            n87 = call-poly <vilib>:"Read Key.vi"("section"=w357, "default value"=u16 0 ("dataProcessor.params.controlFeedback.butterflyValue"), "key"=w355, "refnum"=w356) -> ("value"=w352:u32, "found?"=w362:bool)  [unwired: 4 in, 2 out]
            n88 = call "append default parameters list.vi"("default parameters in"=w358, "parameter found?"=w362, "Key"=w355, "Section"=w357) -> ("default parameters out"=w361:string[])  [unwired: 7 in]
            n89 = Bundle By Name(cluster=w360, "dataProcessor.params.safetyChannels.oilP"=w352) -> (w359:T13)
          }
        }
      }
      frame "fileIO" {
        n90 = case shown="\"startFolder\"" w366 {
          selector: w366 -> [w377 _ w386]
          tunnel: w371 -> [w379 w382 w385]
          tunnel: w370 -> [w378 _ w388]
          tunnel: [w374 w382 w385] -> w369
          tunnel: [w373 w381 w390] -> w368
          tunnel: w367 -> [w373 w381 w391]
          tunnel: [w372 w380 w392] -> w365
          tunnel: w364 -> [w372 w380 w389]
          tunnel: w363 -> [_ _ w387]
          frame "", Default {
            n91 = Concatenate Strings(w378, " : " ("string"), w377) -> (w375:string)
            n92 = Build Array (concatenate)(w379, w375) -> (w374:string[])
          }
          frame "none" {
          }
          frame "startFolder" {
            n93 = call-poly <vilib>:"Read Key.vi"("section"=w388, "default value"=path "C:/Test Data" ("fileIO.params.startFolder"), "key"=w386, "refnum"=w387) -> ("value"=w383:path, "found?"=w393:bool)  [unwired: 4 in, 2 out]
            n94 = call "append default parameters list.vi"("default parameters in"=w389, "parameter found?"=w393, "Key"=w386, "Section"=w388) -> ("default parameters out"=w392:string[])  [unwired: 7 in]
            n95 = Bundle By Name(cluster=w391, "fileIO.params.startFolder"=w383) -> (w390:T13)
          }
        }
      }
      frame "comms" {
        n96 = case shown="\"pulsatorIP\"" w397 {
          selector: w397 -> [w409 _ _ w422 w434 w445 w455 _ w476 _ _]
          tunnel: w403 -> [w411 w414 w418 w426 w438 w449 w459 w468 w480 w487 w493]
          tunnel: w402 -> [w410 _ _ w421 w433 w444 w454 _ w475 _ _]
          tunnel: [w406 w414 w418 w426 w438 w449 w459 w468 w480 w487 w493] -> w401
          tunnel: w400 -> [w405 w413 w420 w429 w440 w451 w462 w470 w482 w489 w495]
          tunnel: [w405 w413 w419 w428 w439 w450 w461 w469 w481 w488 w494] -> w399
          tunnel: w398 -> [_ _ _ w431 w442 w453 w464 _ w483 _ _]
          tunnel: w396 -> [w404 w412 w415 w425 w437 w448 w458 w465 w479 w486 w490]
          tunnel: [w404 w412 w415 w424 w436 w447 w457 w465 w478 w486 w490] -> w395
          tunnel: w394 -> [_ _ w417 _ _ _ _ w467 _ w485 w492]
          frame "", Default {
            n97 = Concatenate Strings(w410, " : " ("string"), w409) -> (w407:string)
            n98 = Build Array (concatenate)(w411, w407) -> (w406:string[])
          }
          frame "none" {
          }
          frame "commandReaderName" {
            n99 = Unbundle By Name(w417) -> ("Comms data.Parameters.command reader name"=w416:string)
            n100 = Bundle By Name(cluster=w420, "comms.params.commandStream.reader name"=w416) -> (w419:T13)
          }
          frame "commandWriterName" {
            n101 = call-poly <vilib>:"Read Key.vi"("section"=w421, "default value"="commandWriter" ("Parameters.error writer name"), "key"=w422, "refnum"=w431) -> ("value"=w427:string, "found?"=w423:bool)  [unwired: 4 in, 2 out]
            n102 = Bundle By Name(cluster=w429, "comms.params.commandStream.writer name"=w427) -> (w428:T13)
            n103 = call "append default parameters list.vi"("default parameters in"=w425, "parameter found?"=w423, "Key"=w422, "Section"=w421) -> ("default parameters out"=w424:string[])  [unwired: 7 in]
          }
          frame "RTIPAddress" {
            n104 = call-poly <vilib>:"Read Key.vi"("section"=w433, "default value"="155.198.87.8" ("Parameters.error writer name"), "key"=w434, "refnum"=w442) -> ("value"=w432:string, "found?"=w435:bool)  [unwired: 4 in, 2 out]
            n105 = Bundle By Name(cluster=w440, "comms.params.RT IP address"=w432, "dataStream.params.Stream.RT IP address"=w432) -> (w439:T13)
            n106 = call "append default parameters list.vi"("default parameters in"=w437, "parameter found?"=w435, "Key"=w434, "Section"=w433) -> ("default parameters out"=w436:string[])  [unwired: 7 in]
          }
          frame "pulsatorIP" {
            n107 = call-poly <vilib>:"Read Key.vi"("section"=w444, "default value"="155.198.87.46" ("Parameters.error writer name"), "key"=w445, "refnum"=w453) -> ("value"=w443:string, "found?"=w446:bool)  [unwired: 4 in, 2 out]
            n108 = Bundle By Name(cluster=w451, "comms.params.pulserControllerIP"=w443) -> (w450:T13)
            n109 = call "append default parameters list.vi"("default parameters in"=w448, "parameter found?"=w446, "Key"=w445, "Section"=w444) -> ("default parameters out"=w447:string[])  [unwired: 7 in]
          }
          frame "errorReaderName" {
            n110 = call-poly <vilib>:"Read Key.vi"("section"=w454, "default value"="errorReader" ("Parameters.error writer name"), "key"=w455, "refnum"=w464) -> ("value"=w460:string, "found?"=w456:bool)  [unwired: 4 in, 2 out]
            n111 = Bundle By Name(cluster=w462, "comms.params.errorStream.reader name"=w460) -> (w461:T13)
            n112 = call "append default parameters list.vi"("default parameters in"=w458, "parameter found?"=w456, "Key"=w455, "Section"=w454) -> ("default parameters out"=w457:string[])  [unwired: 7 in]
          }
          frame "errorWriterName" {
            n113 = Unbundle By Name(w467) -> ("Comms data.Parameters.error writer name"=w466:string)
            n114 = Bundle By Name(cluster=w470, "comms.params.errorStream.writer name"=w466) -> (w469:T13)
          }
          frame "incidentLogfile" {
            w471 = path "C:/Test Data/logfile/test logfile.txt" ("Logfile")
            n115 = call-poly <vilib>:"Read Key.vi"("section"=w475, "default value"=w471, "key"=w476, "refnum"=w483) -> ("value"=w473:path, "found?"=w477:bool)  [unwired: 4 in, 2 out]
            n116 = call "append default parameters list.vi"("default parameters in"=w479, "parameter found?"=w477, "Key"=w476, "Section"=w475) -> ("default parameters out"=w478:string[])  [unwired: 7 in]
            n117 = call "obtain logger queue.vi"() -> ("Incident logger out"=w474:refnum<class "Incident logger.lvclass">)  [unwired: 10 in, 1 out]
            n118 = call "set logfile refnum.vi"("Logfile"=w473, "Incident logger in"=w474) -> ("Incident logger out"=w472:refnum<class "Incident logger.lvclass">)  [unwired: 8 in, 1 out]
            n119 = Bundle By Name(cluster=w482, "comms.vars.Incident logger"=w472, "messageHandler.params.incidentLogfile"=w471) -> (w481:T13)
          }
          frame "commandBufferSize" {
            n120 = Unbundle By Name(w485) -> ("Comms data.Parameters.command buffer size"=w484:i32)
            n121 = Bundle By Name(cluster=w489, "comms.params.commandStream.stream buffer size"=w484) -> (w488:T13)
          }
          frame "errorBufferSize" {
            n122 = Unbundle By Name(w492) -> ("Comms data.Parameters.error buffer size"=w491:i32)
            n123 = Bundle By Name(cluster=w495, "comms.params.errorStream.stream buffer size"=w491) -> (w494:T13)
          }
        }
      }
    }
  }
  "unmatched parameters" <- w21
  "Default parameters" <- w19
  "config parameters" <- w10
  n124 = call <vilib>:"Close Config Data.vi"("write file if changed (T)"=TRUE, "refnum"=w15) -> ()  [unwired: 8 in, 2 out]
  n125 = call "save user config file.vi"("config parameters"=w10) -> ()  [unwired: 11 in]
